vi "Pre Launch Init.vi"(11 "IViewable in":refnum<class "IViewable.lvclass">) -> (0 "error out":errorcluster, 3 "IViewable out":refnum<class "IViewable.lvclass">)   [LabVIEW 2017, in "IViewable.lvlib" / "IViewable.lvclass"]
doc: "(<B>Filename</B>: Actor Framework.lvlib:Actor.lvclass:Pre Launch Init.vi)\n\nDefines behavior that occurs after the Launch Nested Actor method is invoked but before the actor's Actor Core method begins running.\n\nBy default, this method does nothing. A descendant class may override it to define behavior."
uses:
  IViewable.lvclass
  C:/Program Files (x86)/National Instruments/LabVIEW 2017/vi.lib/ActorFramework/Actor/Actor.lvclass
  <vilib>/ActorFramework/Actor/Actor.lvclass/Actor.ctl
  <vilib>/ActorFramework/Message Enqueuer/Message Enqueuer.lvclass/Message Enqueuer.ctl
  <vilib>/ActorFramework/Message Enqueuer/Init from Existing Queue.vi
  <vilib>/ActorFramework/Message Enqueuer/Enqueue.vi
  IViewable Messages/Initialize Front Panel Msg/Initialize Front Panel Msg.lvclass
  C:/Program Files (x86)/National Instruments/LabVIEW 2017/vi.lib/ActorFramework/Message/Message.lvclass
  <vilib>/ActorFramework/Message Priority Queue/Priority Enqueue.vi
  ActorEvents/IEventAggregator/IEventAggregator.lvclass
  <vilib>/ActorFramework/Message Enqueuer/Message Enqueuer.lvclass
  <vilib>/ActorFramework/Actor/Actor.lvclass
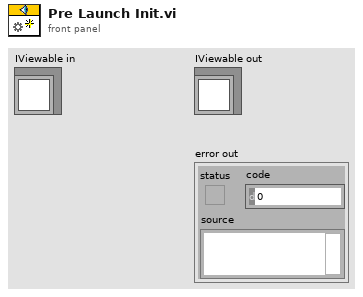
[diagram p1: front panel]
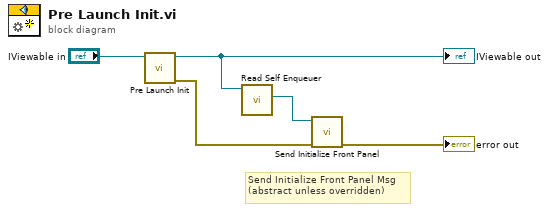
[diagram p0: block diagram]
diagram:
  # "Send Initialize Front Panel Msg\n(abstract unless overridden)"
  n1 = call-parent "Pre Launch Init.vi"("IEventAggregator in"="IViewable in") -> ("error out"=w5:errorcluster, "IEventAggregator out"=w3:refnum<class "IViewable.lvclass">)  [unwired: 9 in]
  "IViewable out" <- w3
  n2 = call <vilib>:"Read Self Enqueuer.vi"("Actor"=w3) -> ("Self Enqueuer"=w1:refnum<class "Message Enqueuer.lvclass">)  [unwired: 10 in]
  n3 = call "Send Initialize Front Panel.vi"("error in (no error)"=w5, "Message Enqueuer"=w1) -> ("error out"=→"error out":errorcluster)  [unwired: 8 in, 1 out]
